vi "Close_unit.vi"(8 "error in (no error)":errorcluster, 11 "Handle":i16) -> (0 "error out":errorcluster)   [LabVIEW 2023]
uses:
  ps2000.dll
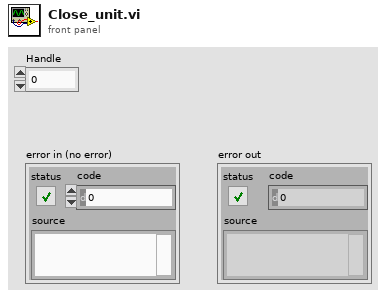
[diagram p1: front panel]
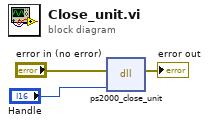
[diagram p0: block diagram]
diagram:
  n1 = dll-call lib="C:/Users/cesar/Desktop/Ps2000 libreria/PS2000.dll" fn="ps2000_close_unit"(error in="error in (no error)", "Handle"="Handle") -> (error out=→"error out":errorcluster)  [unwired: 4 in, 1 out]
